vi "DaxsonicsBP2.vi"(11 "Uniform Gain":bool=TRUE) -> ()   [LabVIEW 2022 SP3]
doc: "This application VI allows the user to set the desired parameters in the Daxsonics BP2"
uses:
  ScanningControl/Motion Controllers/-MotionRoutines/MotionGlobals.vi
panel:
  in  "Freq (MHz)":u16(ring)=20 items=["4"=4, "6"=6, "8"=8, "10"=10, "12"=12, "15"=15, "17"=17, "20"=20, "25"=25, "30"=30, "35"=35, "40"=40, "45"=45, "50"=50]
  in  "Gains":u16[](array[ring]) items=["22"=22, "25"=25, "28"=28, "31"=31, "34"=34, "37"=37, "40"=40, "43"=43, "46"=46, "49"=49, "52"=52, "55"=55, "58"=58, "61"=61, "64"=64]
  in  "Amp (V)":u16(ring) items=["0"=0, "10"=10, "20"=20, "30"=30, "40"=40, "50"=50, "60"=60, "70"=70, "80"=80, "90"=90, "100"=100, "110"=110, "120"=120, "130"=130, "140"=140, "150"=150, "160"=160, "170"=170, "180"=180, "190"=190]
  in  "Lock/Unlock":bool
  in  "ExitSendCmd":bool
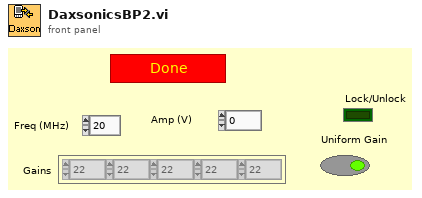
[diagram p1: front panel]
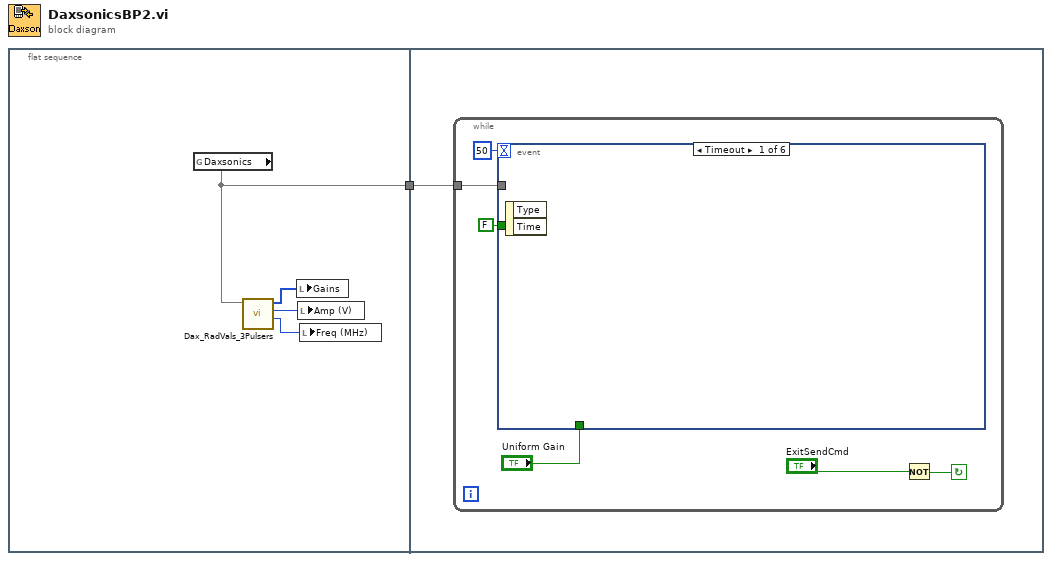
[diagram p0: block diagram]
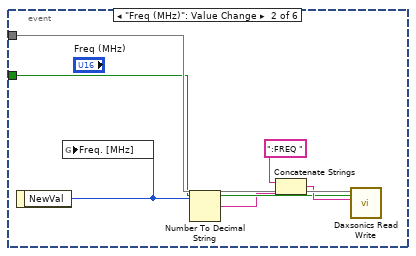
[diagram p2: hidden frame]
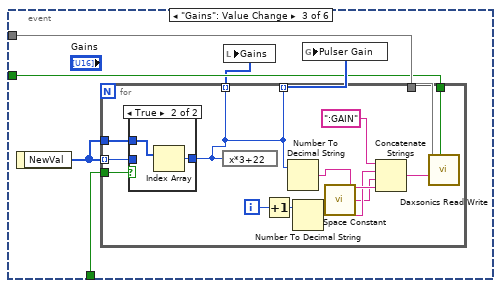
[diagram p3: hidden frame]
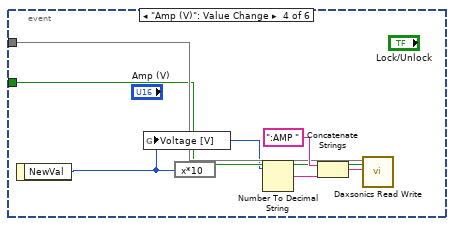
[diagram p5: hidden frame]
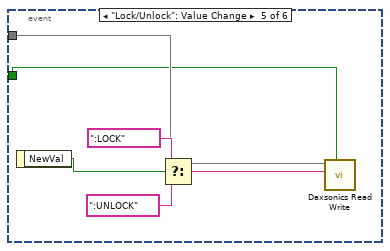
[diagram p6: hidden frame]
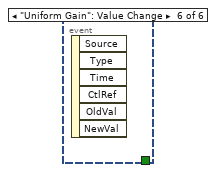
[diagram p7: hidden frame]
diagram:
  n1 = flat-sequence {
    tunnel: [w5] -> w1
    tunnel: w1 -> [w6]
    frame #0 {
      n2 = global read "MotionGlobals.vi" "Daxsonics"() -> (w5)
      n3 = call "Dax_RadVals_3Pulsers.vi"("Daxsonics"=w5) -> ("Freq (MHz)"=w4:u16, "Voltage (V)"=w3:u16, "Gains"=w2:u16[])  [unwired: 7 in, 1 out]
      n4 = local write "Gains"(w2) -> ()
      n5 = local write "Amp (V)"(w3) -> ()
      n6 = local write "Freq (MHz)"(w4) -> ()
    }
    frame #1 {
      n7 = while {
        tunnel: w6 -> [w9]
        stop <- w12 continue-if-true
        n8 = event shown="[0] Timeout" {
          selector: _ -> [_ _ _ _ _ _]
          dyn-events: _ -> [_ _ _ _ _ _]
          timeout: 50 -> [_ _ _ _ _ _]
          tunnel: w9 -> [_ w17 w24 w43 w48 _]
          tunnel: FALSE ("Enable Termination\nChar (T)") -> [_ w15 w22 w42 w47 _]
          tunnel: "Uniform Gain" -> [_ _ w21 _ _ _]
          event Timeout {
            n9 = event-data() -> ()  [unwired: 3 out]
          }
          event "Freq (MHz)": Value Change {
            n10 = event-data() -> ("NewVal"=w13:u16)  [unwired: 1 out]
            n11 = global write "MotionGlobals.vi" "Freq. [MHz]"(w13) -> ()
            n12 = Number To Decimal String(number=w13) -> (decimal integer string=w14:string)  [unwired: 1 in]
            n13 = Concatenate Strings(":FREQ " ("string"), w14) -> (w16:string)
            n14 = call "Daxsonics Read Write.vi"("Daxsonics Name"=w15, "write buffer"=w16, "VISA resource name"=w17) -> ()  [unwired: 6 in, 3 out]
          }
          event "Gains": Value Change {
            n15 = event-data() -> ("NewVal"=w20:u16[])  [unwired: 1 out]
            n16 = for {
              tunnel: w20 -> [w28] mode=indexing
              tunnel: w24 -> [w34]
              tunnel: [w25] -> w23 mode=indexing
              tunnel: w22 -> [w30]
              tunnel: w21 -> [w27]
              tunnel: w20 -> [w26]
              tunnel: [w25] -> w19 mode=indexing
              i -> [w33]
              n17 = case shown="True" w27 {
                tunnel: w28 -> [w38 _]
                tunnel: [w38 w39] -> w25
                tunnel: w26 -> [_ w40]
                frame False {
                }
                frame True {
                  n18 = Index Array(array=w40) -> (element=w39:u16)  [unwired: 1 in]
                }
              }
              n19 = expression code="x*3+22"(w25) -> ()  [unwired: 1 out]
              n20 = Increment(x=w33) -> (x+1=w29:i32)
              n21 = Number To Decimal String(number=w25) -> (decimal integer string=w37:string)  [unwired: 1 in]
              n22 = Number To Decimal String(number=w29) -> (decimal integer string=w32:string)  [unwired: 1 in]
              n23 = call <vilib>:"Space Constant.vi"() -> ("String"=w31:string)
              n24 = Concatenate Strings(":GAIN" ("string"), w32, w31, w37) -> (w36:string)
              n25 = call "Daxsonics Read Write.vi"("Daxsonics Name"=w30, "write buffer"=w36, "VISA resource name"=w34) -> ()  [unwired: 6 in, 3 out]
            }
            n26 = local write "Gains"(w19) -> ()
            n27 = global write "MotionGlobals.vi" "Pulser Gain"(w23) -> ()
          }
          event "Amp (V)": Value Change {
            n28 = event-data() -> ("NewVal"=w41:u16)  [unwired: 1 out]
            n29 = global write "MotionGlobals.vi" "Voltage [V]"(w41) -> ()
            n30 = expression code="x*10"(w41) -> ()  [unwired: 1 out]
            n31 = Number To Decimal String(number=w41) -> (decimal integer string=w46:string)  [unwired: 1 in]
            n32 = Concatenate Strings(":AMP " ("string"), w46) -> (w45:string)
            n33 = call "Daxsonics Read Write.vi"("Daxsonics Name"=w42, "write buffer"=w45, "VISA resource name"=w43) -> ()  [unwired: 6 in, 3 out]
          }
          event "Lock/Unlock": Value Change {
            n34 = event-data() -> ("NewVal"=w52:bool)  [unwired: 1 out]
            n35 = Select(t=":LOCK", s=w52, f=":UNLOCK") -> (s? t:f=w49:string)
            n36 = call "Daxsonics Read Write.vi"("Daxsonics Name"=w47, "write buffer"=w49, "VISA resource name"=w48) -> ()  [unwired: 6 in, 3 out]
          }
          event "Uniform Gain": Value Change {
            n37 = event-data() -> ()  [unwired: 7 out]
          }
        }
        n38 = Not(x="ExitSendCmd") -> (.not. x?=w12:bool)
      }
    }
  }
